vi "DSF.Shared.Configuration.Get Settings.vi"(11 "Configuration in":refnum<class "DSF.Shared.Configuration.lvclass">) -> (2 "settings":T1, 3 "Configuration out":refnum<class "DSF.Shared.Configuration.lvclass">)   [LabVIEW 2017, in "DSF.Engine.lvlib" / "DSF.Shared.Configuration.lvclass"]
uses:
  DSF.Shared.Configuration.lvclass
  DSF Configuration API/1.0.0/Public/Controls/DSF Settings Info.ctl
  DSF.Shared.Configuration.lvclass/DSF.Shared.Configuration.ctl
  DSF Configuration API/1.0.0/DSF Configuration API.lvlib
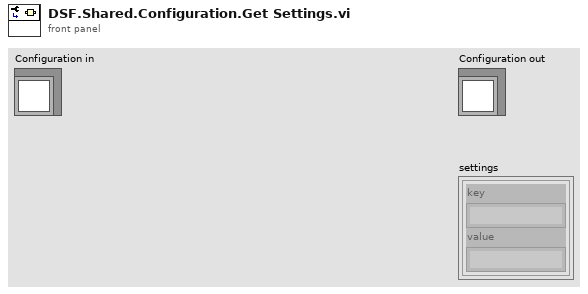
[diagram p1: front panel]
types:
  T1 = typedef "DSF Configuration API.lvlib/DSF Settings Info.ctl" = cluster{"key":string, "value":string}[]
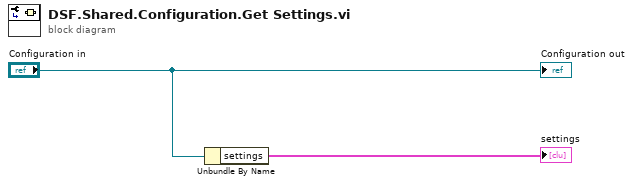
[diagram p0: block diagram]
diagram:
  n1 = Unbundle By Name("Configuration in") -> ("settings"=→"settings":T1)
  "Configuration out" <- "Configuration in"
